vi "Assert No Driver Error.vi"(8 "error in":errorcluster, 11 "driver vi name":string="Self Test") -> (0 "error out":errorcluster, 2 "result":string, 3 "pass?":bool)   [LabVIEW 2020, in "MeasurementServerTests.lvlib"]
uses:
  MeasurementServerTests.lvlib
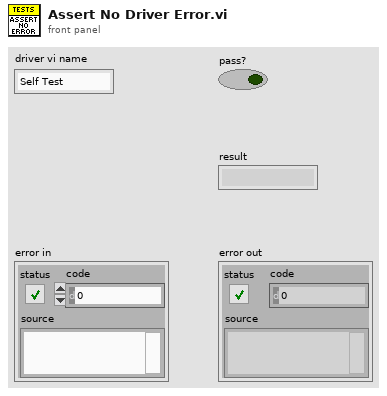
[diagram p1: front panel]
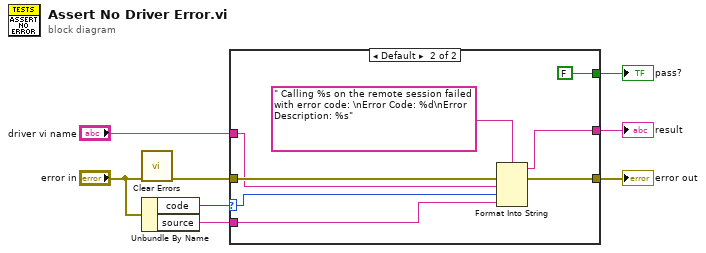
[diagram p0: block diagram]
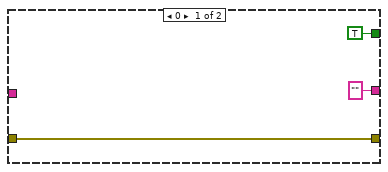
[diagram p2: hidden frame]
diagram:
  n1 = call <vilib>:"Clear Errors.vi"("error in (no error)"="error in") -> ("error out"=w3:errorcluster)  [unwired: 5 in, 1 out]
  n2 = Unbundle By Name("error in") -> ("code"=w4:i32, "source"=w1:string)
  n3 = case shown="Default" w4 {
    selector: w4 -> [_ w14]
    tunnel: ["" w18] -> w7
    tunnel: [TRUE FALSE] -> w6
    tunnel: w3 -> [w10 w16]
    tunnel: [w10 w15] -> w8
    tunnel: "driver vi name" -> [_ w13]
    tunnel: w1 -> [_ w12]
    frame 0 {
    }
    frame Default {
      n4 = Format Into String(format string=" Calling %s on the remote session failed with error code: \nError Code: %d\nError Description: %s" ("f"), error in=w16, w13, w14, w12) -> (resulting string=w18:string, error out=w15:errorcluster)  [unwired: 1 in]
    }
  }
  "error out" <- w8
  "result" <- w7
  "pass?" <- w6
